vi "SSD1306_DrawProgress.vi"(8 "error in (no error)":errorcluster, 10 "percentage":u8, 11 "String":string) -> (0 "error out":errorcluster)   [LabVIEW 2014, in "QwaveSys_Interface.lvlib"]
uses:
  QwaveSys_Interface.lvlib
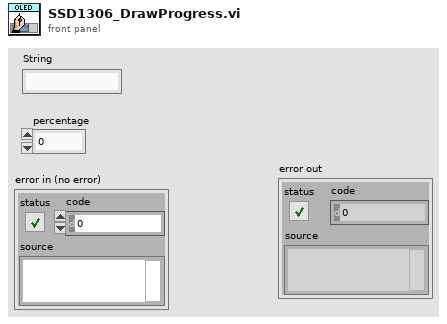
[diagram p1: front panel]
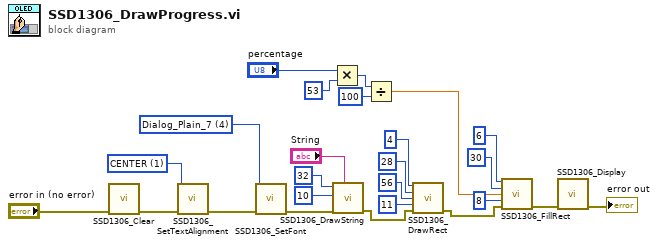
[diagram p0: block diagram]
diagram:
  w1 = u16 4 items=["Calligraffitti_Plain_10", "ArialMT_Plain_10", "ArialMT_Plain_16", "ArialMT_Plain_24", "Dialog_Plain_7"] ("Font")
  w21 = u16 1 items=["LEFT", "CENTER", "RIGHT"] ("alignment")
  n1 = call "SSD1306_Clear.vi"("error in (no error)"="error in (no error)") -> ("error out"=w25:errorcluster)  [unwired: 10 in]
  n2 = call "SSD1306_SetTextAlignment.vi"("error in (no error)"=w25, "alignment"=w21) -> ("error out"=w20:errorcluster)  [unwired: 9 in]
  n3 = call "SSD1306_SetFont.vi"("error in (no error)"=w20, "Font"=w1) -> ("error out"=w18:errorcluster)  [unwired: 9 in]
  n4 = Multiply(x="percentage", y=u32 53 ("width")) -> (x*y=w5:u32)
  n5 = call "SSD1306_DrawString.vi"("String"="String", "error in (no error)"=w18, "y"=u8 10, "x"=u8 32) -> ("error out"=w11:errorcluster)  [unwired: 7 in]
  n6 = Divide(x=w5, y=u8 100) -> (x/y=w3:dbl)
  n7 = call "SSD1306_DrawRect.vi"("x"=u8 4, "y"=u8 28, "width"=u8 56, "height"=u8 11, "error in (no error)"=w11) -> ("error out"=w16:errorcluster)  [unwired: 10 in]
  n8 = call "SSD1306_FillRect.vi"("x"=u8 6, "y"=u8 30, "width"=w3, "height"=u8 8, "error in (no error)"=w16) -> ("error out"=w10:errorcluster)  [unwired: 10 in]
  n9 = call "SSD1306_Display.vi"("error in (no error)"=w10) -> ("error out"=→"error out":errorcluster)  [unwired: 10 in]
